vi "SIAM-Connectiontest.vi"() -> ()   [LabVIEW 2011]
panel:
  out "length":i32=64
  out "data out 4":string
  out "data out 3":string
  in  "ZNQ minimal 4":string="ÿ\u0000\u0000\u0000\u0000\u0000\u0000\u0000\u0001\u0000"
  in  "ZNQ i am V2":string="ÿ\u0000\u0000\u0000\u0000\u0000\u0000\u0000\u0000\u0002"
  out "data out 2":string
  in  "ZNQ minimal 2":string="ÿ\u0000\u0000\u0000\u0000\u0000\u0000\u0000\u0000"
  out "OK response12byte":string
  in  "bytes to read":i32=64
  in  "ZNQ minimal":string="ÿ\u0000\u0000\u0000\u0000\u0000\u0000\u0000\u0001\u0003\u0001HELLO me 123"
  in  "Port3 message pwd till-x-4":string="\u0000\u0000\u0000\n\u0000\u0000\u0000I\u0000\u0000\u0000\u0000\u0000\u0000\u0000t\u0000\u0000\u0000i\u0000\u0000\u0000l\u0000\u0000\u0000l\u0000\u0000\u0000-\u0000\u0000\u0000x\u0000\u0000\u0000-\u0000\u0000\u00004"
  out "error out":errorcluster
  out "write":errorcluster
  out "connect":errorcluster
  out "bytes written":i32=24
  out "read":errorcluster
  out "data out":string
  in  "remote port":u16=9912
  in  "address":string="10.10.2.104"
  # "https://rfc.zeromq.org/spec/24/"
  # "F\\03  > Version3"
  # "???\n10 with ZMTP/1\n11 with ZMTP/2"
  # "wrong IP connect errror 56"
  # "+ getting"
  # "01\\7F\\xx"
  # "correct IP, wrong port\nsiam:3 wrong pwd: read error 56: time out  0,0,56,0\nsiam:9912,9913: \"till-x-4: err 66, connection closed 0,0,66,0\nsiam 9914: connect 56: time out   56,56,1,1"
  # "expect  return\n2,49,0\n49,AE =Wrong Password"
  # "greeding 64octets"
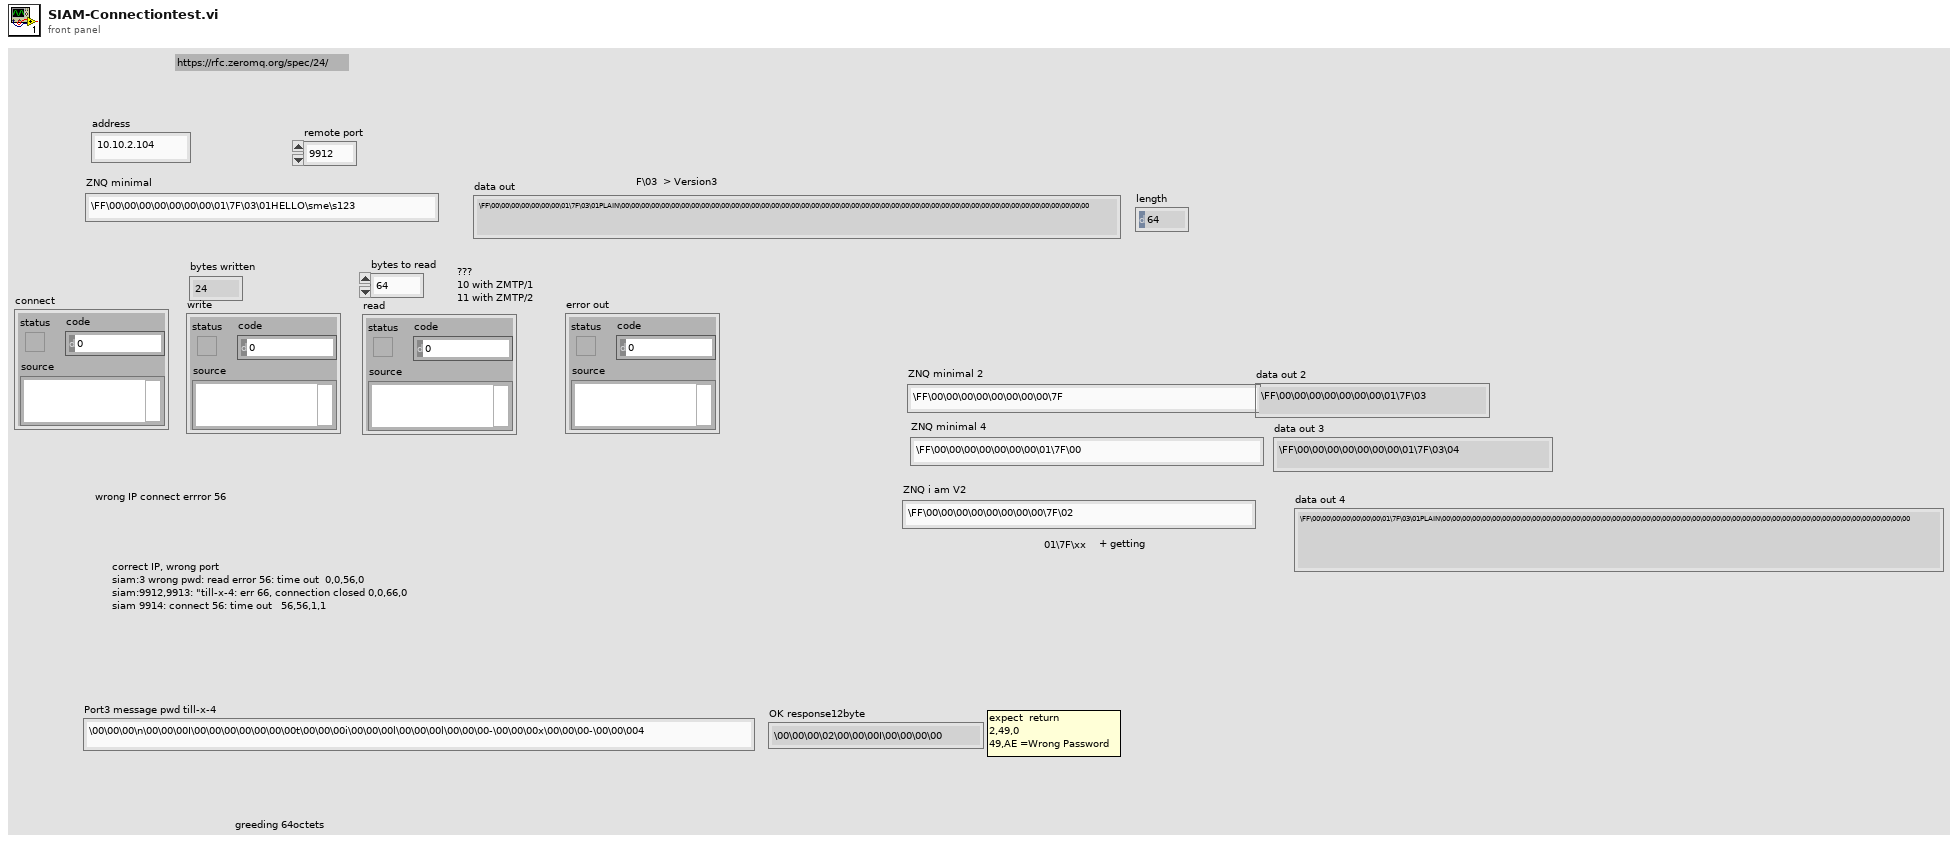
[diagram p1: front panel]
types:
  T1 = enum16{"Standard", "Buffered", "CRLF", "Immediate"}
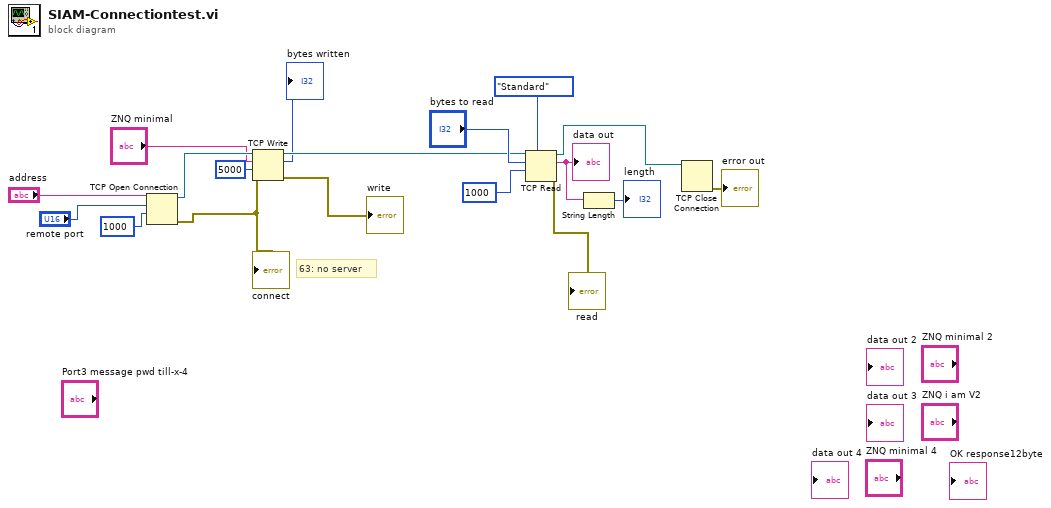
[diagram p0: block diagram]
diagram:
  # "63: no server"
  n1 = TCP Open Connection(address="address", remote port or service name="remote port", timeout ms (60000)=1000) -> (connection ID=w18:refnum<k5>, error out=w13:errorcluster)  [unwired: 1 in, 1 out]
  "connect" <- w13
  n2 = TCP Write(connection ID=w18, data in="ZNQ minimal", error in (no error)=w13, 9:5000 ("timeout ms (25000)")) -> (connection ID out=w9:refnum<k5>, bytes written=→"bytes written":i32, error out=→"write":errorcluster)
  n3 = TCP Read(connection ID=w9, bytes to read="bytes to read", 7:T1."Standard" ("mode (standard)"), 9:1000 ("timeout ms (25000)")) -> (connection ID out=w7:refnum<k5>, data out=w2:string, error out=→"read":errorcluster)  [unwired: 1 in]
  "data out" <- w2
  n4 = String Length(string=w2) -> (length=→"length":i32)
  n5 = TCP Close Connection(connection ID=w7) -> (error out=→"error out":errorcluster)  [unwired: 1 in, 2 out]
